vi "Read.vi"(8 "error in":errorcluster, 11 "Chiller Cluster - 1 Channel.lvclass":refnum<class "Chiller Cluster - 1 Channel.lvclass">) -> (0 "error out":errorcluster, 3 "output cluster":refnum<class "Chiller Cluster - 1 Channel.lvclass">)   [LabVIEW 2023, in "Chiller Cluster - 1 Channel.lvclass"]
uses:
  Chiller Cluster - 1 Channel.lvclass
  Chiller Cluster - 1 Channel.lvclass/Chiller Cluster - 1 Channel.ctl
  ef93f7cc-46a7-4415-853b-c3da1f88e6bb.vi
  9c8d422d-920d-4f62-ba29-e6a76558d5ae.vi
  ef93f7cc-46a7-4415-853b-c3da1f88e6bb.vi/c28b0ead-42ad-4072-80a2-aca7f2bd7ce3.vi
  ef93f7cc-46a7-4415-853b-c3da1f88e6bb.vi/219d0231-d98b-4193-b5cc-84f90e3c9091.vi
  9c8d422d-920d-4f62-ba29-e6a76558d5ae.vi/c28b0ead-42ad-4072-80a2-aca7f2bd7ce3.vi
  9c8d422d-920d-4f62-ba29-e6a76558d5ae.vi/219d0231-d98b-4193-b5cc-84f90e3c9091.vi
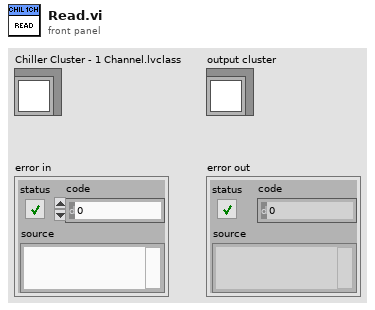
[diagram p1: front panel]
types:
  T1 = cluster{"OnOff.ACT":bool, "ErrorAcknowledge.ACT":bool}
  T2 = cluster{"ErrorAcknowledge.ch01.ACT":bool, "OutputEnable.ch01.ACT":bool, "ControlMode.ch01.CTL":u16, "Temperature.ch01.SP":dbl, "TemperatureMIN.ch01.SP":dbl, "TemperatureMAX.ch01.SP":dbl, "TemperatureGrad.ch01.SP":dbl, "Pressure.ch01.SP":dbl, "PressureMIN.ch01.SP":dbl, "PressureMAX.ch01.SP":dbl, "PressureGrad.ch01.SP":dbl, "Flow.ch01.SP":dbl, "FlowMIN.ch01.SP":dbl, "FlowMAX.ch01.SP":dbl, "FlowGrad.ch01.SP":dbl}
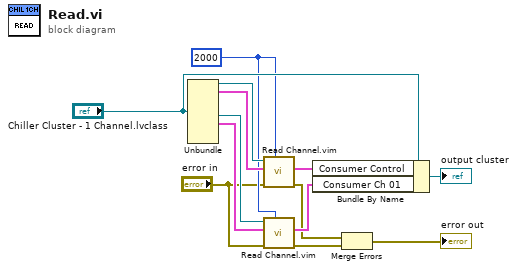
[diagram p0: block diagram]
diagram:
  w8 = 2000 ("Timeout (ms)")
  n1 = Unbundle("Chiller Cluster - 1 Channel.lvclass") -> (w10:refnum<k21>, w9:T1, w7:refnum<k21>, w6:T2)  [unwired: 4 out]
  n2 = call "Read Channel.vim"("Timeout (ms)"=w8, "error in"="error in", "Data in"=w9, "ADAS HIL Channel in"=w10) -> ("error out"=w3:errorcluster, "Data out"=w11:T1)  [unwired: 4 in, 2 out]
  n3 = call "Read Channel.vim"("Timeout (ms)"=w8, "error in"="error in", "Data in"=w6, "ADAS HIL Channel in"=w7) -> ("error out"=w2:errorcluster, "Data out"=w5:T2)  [unwired: 4 in, 2 out]
  n4 = Bundle By Name(cluster="Chiller Cluster - 1 Channel.lvclass", "Consumer Control"=w11, "Consumer Ch 01"=w5) -> (→"output cluster":refnum<class "Chiller Cluster - 1 Channel.lvclass">)
  n5 = Merge Errors(w3, w2) -> (→"error out":errorcluster)
